vi "Initialize.vi"(8 "error in (no error)":errorcluster, 10 "Top Level Diagram":refnum<vi>, 11 "IO Loop in":refnum<class "Module Loop.lvclass">) -> (0 "error out":errorcluster, 3 "IO Loop out":refnum<class "Module Loop.lvclass">)   [LabVIEW 2015, in "Module Loop.lvclass"]
uses:
  Module Loop.lvclass
  Structures/Structures.lvclass
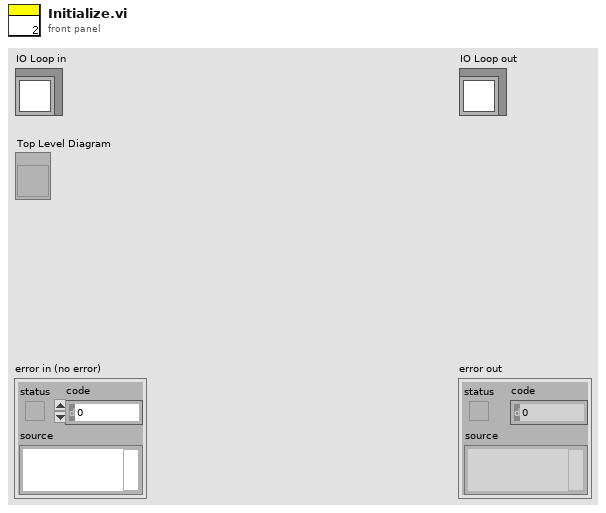
[diagram p1: front panel]
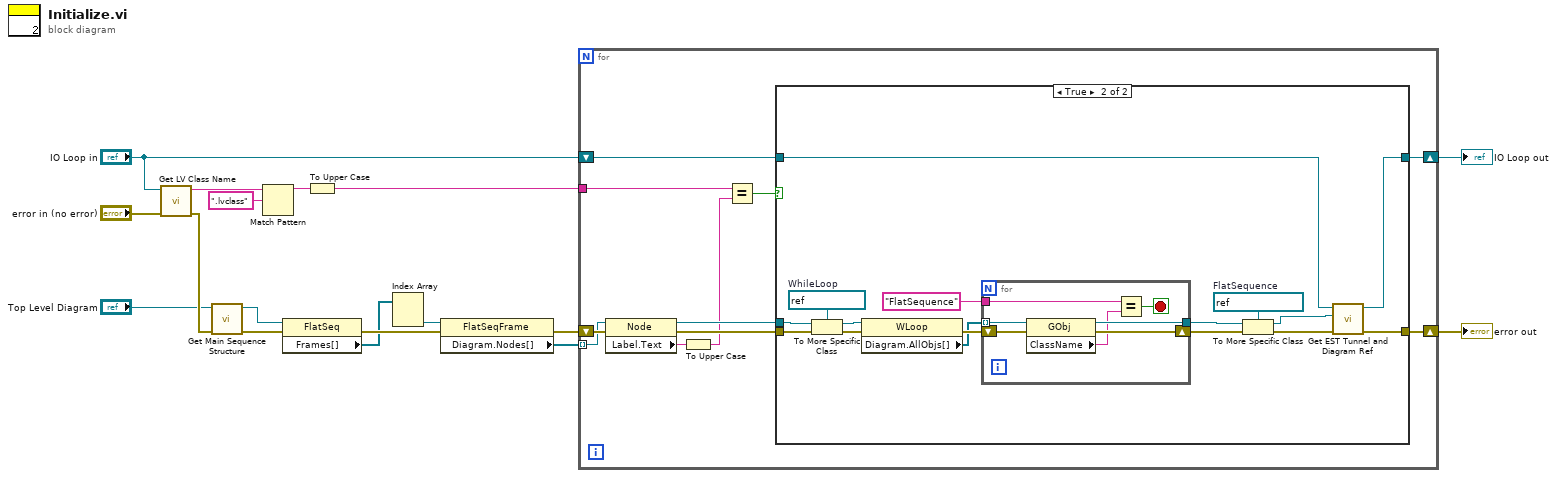
[diagram p0: block diagram]
diagram:
  n1 = call <vilib>:"Get LV Class Name.vi"("error in (no error)"="error in (no error)", "object"="IO Loop in") -> ("error out"=w7:errorcluster, "class name"=w12:string)  [unwired: 8 in]
  n2 = call "Get Main Sequence Structure.vi"("error in (no error)"=w7, "Top Level Diagram"="Top Level Diagram") -> ("error out"=w6:errorcluster, "Main.SeqStructure"=w5:refnum<vi>)  [unwired: 8 in]
  n3 = Match Pattern(string=w12, regular expression=".lvclass") -> (before substring=w10:string)  [unwired: 1 in, 3 out]
  n4 = property class="FlatSeq"(reference=w5, error in=w6) -> (error out=w14:errorcluster, "Frames[]"=w13:refnum<vi>[])  [unwired: 1 out]
  n5 = To Upper Case(1:w10) -> (0:w9:string)
  n6 = Index Array(array=w13) -> (element #2=w17:refnum<vi>)  [unwired: 2 in, 1 out]
  n7 = property class="FlatSeqFrame"(reference=w17, error in=w14) -> (error out=w16:errorcluster, "Diagram.Nodes[]"=w15:refnum<vi>[])  [unwired: 1 out]
  n8 = for {
    tunnel: w15 -> [w27] mode=indexing
    shift-right: [w23] -> w8
    shift-left: w16 -> [w28]
    tunnel: w9 -> [w21]
    shift-right: [w19] -> w1
    shift-left: "IO Loop in" -> [w20]
    n9 = property class="Node"(reference=w27, error in=w28) -> (reference out=w25:refnum<vi>, error out=w24:errorcluster, "Label.Text"=w26:string)
    n10 = To Upper Case(1:w26) -> (0:w22:string)
    n11 = Equal?(x=w21, y=w22) -> (x = y?=w18:bool)
    n12 = case shown="True" w18 {
      tunnel: w25 -> [_ w45]
      tunnel: w24 -> [w30 w46]
      tunnel: [w30 w32] -> w23
      tunnel: w20 -> [w29 w33]
      tunnel: [w29 w31] -> w19
      frame False {
      }
      frame True {
        w44 = refnum<vi> refnum  # WhileLoop
        w38 = refnum<vi> refnum  # FlatSequence
        n13 = To More Specific Class(target class=w44, reference=w45, error in=w46) -> (specific class reference=w43:refnum<vi>, error out=w42:errorcluster)
        n14 = property class="WLoop"(reference=w43, error in=w42) -> (error out=w41:errorcluster, "Diagram.AllObjs[]"=w40:refnum<vi>[])  [unwired: 1 out]
        n15 = for {
          shift-right: [w52] -> w39
          shift-left: w41 -> [w53]
          tunnel: w40 -> [w51] mode=indexing
          tunnel: "FlatSequence" ("name/order") -> [w50]
          tunnel: [w48] -> w36
          stop <- w49 stop-if-true
          n16 = property class="GObj"(reference=w51, error in=w53) -> (reference out=w48:refnum<vi>, error out=w52:errorcluster, "ClassName"=w47:string)
          n17 = Equal?(x=w50, y=w47) -> (x = y?=w49:bool)
        }
        n18 = To More Specific Class(target class=w38, reference=w36, error in=w39) -> (specific class reference=w34:refnum<vi>, error out=w35:errorcluster)
        n19 = call-dynamic "Get EST Tunnel and Diagram Ref.vi"("error in (no error)"=w35, "FlatSeq Refnum"=w34, "IO Loop in"=w33) -> ("error out"=w32:errorcluster, "IO Loop out"=w31:refnum<class "Module Loop.lvclass">)  [unwired: 7 in]
      }
    }
  }
  "error out" <- w8
  "IO Loop out" <- w1
